vi "VISA MEMACC Write U8 vs U64.vi"() -> ()   [LabVIEW 2016]
uses:
  <vilib>/Platform/TimedLoop/XDataNode/timing_clust.ctl
  <vilib>/Platform/TimedLoop/XDataNode/nitl_modes.ctl
  <vilib>/Platform/TimedLoop/XDataNode/wakeup.ctl
  Source/GE 5565PIORC/GE 5565PIORC.lvclass/GE 5565PIORC.ctl
  Source/GE 5565PIORC/VIs/Block Operations/Allocate Single Block.vi
  Source/GE 5565PIORC/VIs/Registers/Local Configuration.LAS1RR.Address Range.Get.vi
  Source/GE 5565PIORC/VIs/Binary Operations/Align to 8-byte Boundary.vi
  Source/GE 5565PIORC/VIs/Binary Operations/Align to 16-byte Boundary.vi
  Source/GE 5565PIORC/VIs/Registers/Local Configuration.Get Register Offset.vi
  Source/GE 5565PIORC/GE 5565PIORC.lvclass
  <vilib>/platform/TimedLoop/XDataNode/XDataNode.xnode
  <vilib>/Platform/TimedLoop/XDataNode/XDNodeRunTimeDep.lvlib
panel:
  out "U64 Duration":dbl
  in  "U64s":i32
  out "U8 Duration":dbl
  in  "VISA resource name":refnum<visa-resource-name>
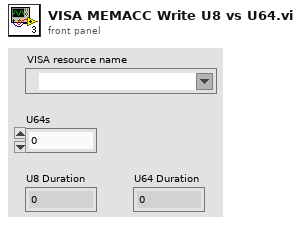
[diagram p1: front panel]
types:
  T1 = typedef "XDNodeRunTimeDep.lvlib/timing_clust.ctl" = cluster{"Expected End [f-1]":u64, "Actual End [f-1]":u64, "Finished Late? [f-1]":bool, "Expected End [i-1]":u64, "Actual End [i-1]":u64, "Finished Late? [i-1]":bool, "Expected Start [i]":u64, "Actual Start [i]":u64, "Expected Start [f]":u64, "Actual Start [f]":u64, "Source Name":string, "Structure Name":string, "Period":i64, "Deadline":i64, "Offset":i64, "Start":i64, "Priority":i32, "Timeout":i32, "Mode":T2, "Wakeup Reason":T3, "Error":errorcluster, "Source Type":string, "Secondary Source Type":string, "Global End Time":u64, "Global Start Time":u64, "Frame Duration":u64, "Iteration Duration":u64, "Assigned CPU":i32, "I/O Scan Engine Mode":u32}
  T2 = typedef "XDNodeRunTimeDep.lvlib/nitl_modes.ctl" = enum32{"No Change", "Process missed periods, maintain original phase", "Discard missed periods, maintain original phase", "Process missed periods, ignore original phase", "Discard missed periods, ignore original phase"}
  T3 = typedef "XDNodeRunTimeDep.lvlib/wakeup.ctl" = enum32{"Normal", "Aborted", "Asynchronous wakeup", "Timing source error", "Timed loop error", "Timeout"}
  T4 = typedef "GE 5565PIORC.lvclass/DMA Block Descriptor.ctl" = cluster{"descriptor ptr (VISA)":u32, "descriptor size":u32, "descriptor ptr (aligned)":u32, "data ptr (lower)":u32, "data ptr (upper)":u32, "data size":u32, "next descriptor ptr":u32}
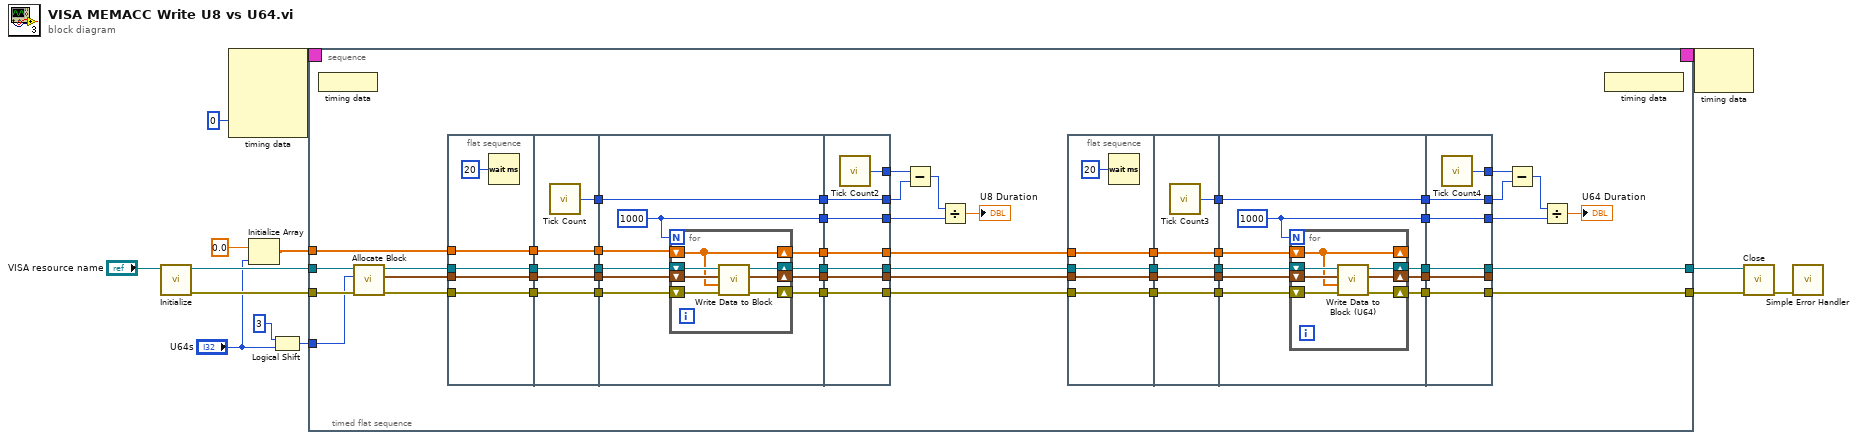
[diagram p0: block diagram]
diagram:
  n1 = call "Initialize.vi"("VISA resource name"="VISA resource name") -> ("error out"=w8:errorcluster, "GE 5565PIORC"=w9:refnum<class "GE 5565PIORC.lvclass">)  [unwired: 9 in]
  n2 = node-c288(0 ("Processor")) -> (w12:T1)  [unwired: 3 in]
  n3 = Initialize Array(0.0 ("element"), "U64s") -> (w1:dbl[])
  n4 = Logical Shift(y=i16 3, x="U64s") -> (x << y=w7:i32)
  n5 = timed-sequence {
    timing: w12 -> [_]
    timing-out: [_] -> w11
    tunnel: w9 -> [w17]
    tunnel: w8 -> [w20]
    tunnel: [w19] -> w4
    tunnel: w7 -> [w18]
    tunnel: [w16] -> w5
    tunnel: w1 -> [w15]
    n6 = timed-flat-sequence {
      tunnel: w20 -> [w45]
      tunnel: [w47] -> w19
      tunnel: w18 -> [w42]
      tunnel: w17 -> [w46]
      tunnel: [w28] -> w16
      tunnel: w15 -> [w27]
      n7 = node-c288() -> ()  [unwired: 1 in]
      n8 = call-poly "Allocate Block.vi"("error in (no error)"=w45, "size (bytes)"=w42, "GE 5565PIORC in"=w46) -> ("error out"=w43:errorcluster, "Block Descriptor"=w37:T4, "GE 5565PIORC out"=w44:refnum<class "GE 5565PIORC.lvclass">)  [unwired: 6 in]
      n9 = flat-sequence {
        tunnel: w44 -> [w108]
        tunnel: w43 -> [w107]
        tunnel: [w108] -> w67
        tunnel: [w107] -> w65
        tunnel: w37 -> [w106]
        tunnel: [w106] -> w36
        tunnel: w27 -> [w105]
        tunnel: [w105] -> w26
        tunnel: [w114] -> w72
        tunnel: [w113] -> w68
        tunnel: w67 -> [w113]
        tunnel: [w112] -> w66
        tunnel: w65 -> [w112]
        tunnel: w36 -> [w111]
        tunnel: [w111] -> w35
        tunnel: w26 -> [w110]
        tunnel: [w110] -> w25
        tunnel: w72 -> [w124]
        tunnel: [w124] -> w71
        tunnel: w68 -> [w121]
        tunnel: w66 -> [w120]
        tunnel: [w123] -> w64
        tunnel: [w122] -> w63
        tunnel: [w119] -> w41
        tunnel: w35 -> [w118]
        tunnel: [w117] -> w34
        tunnel: w25 -> [w116]
        tunnel: [w115] -> w24
        tunnel: [w138] -> w70
        tunnel: [w137] -> w69
        tunnel: w71 -> [w137]
        tunnel: w64 -> [w136]
        tunnel: [w136] -> w48
        tunnel: w63 -> [w135]
        tunnel: [w135] -> w61
        tunnel: w41 -> [w134]
        tunnel: [w134] -> w38
        tunnel: w34 -> [w133]
        tunnel: [w133] -> w33
        tunnel: w24 -> [w132]
        tunnel: [w132] -> w23
        frame #0 {
          n10 = Wait (ms)(milliseconds to wait=u32 20) -> ()  [unwired: 1 out]
        }
        frame #1 {
          n11 = call "Tick Count"() -> ("Tick Count(uSec)"=w114:u32)
        }
        frame #2 {
          w122 = 1000
          n12 = for {
            N: w122 -> [_]
            shift-right: [w130] -> w119
            shift-left: w121 -> [w131]
            shift-right: [w128] -> w123
            shift-left: w120 -> [w129]
            shift-right: [w127] -> w117
            shift-left: w118 -> [w126]
            shift-right: [w125] -> w115
            shift-left: w116 -> [w125]
            n13 = call "Write Data to Block.vi"("error in (no error)"=w129, "Data"=w125, "Block Descriptor"=w126, "GE 5565PIORC"=w131) -> ("error out"=w128:errorcluster, "Block Descriptor out"=w127:T4, "GE 5565PIORC out"=w130:refnum<class "GE 5565PIORC.lvclass">)  [unwired: 5 in]
          }
        }
        frame #3 {
          n14 = call "Tick Count2"() -> ("Tick Count(uSec)"=w138:u32)
        }
      }
      n15 = Subtract(x=w70, y=w69) -> (x-y=w62:u32)
      n16 = Divide(x=w62, y=w61) -> (x/y=→"U8 Duration":dbl)
      n17 = flat-sequence {
        tunnel: w48 -> [w76]
        tunnel: [w76] -> w59
        tunnel: [w75] -> w39
        tunnel: w38 -> [w75]
        tunnel: w33 -> [w74]
        tunnel: [w74] -> w32
        tunnel: w23 -> [w73]
        tunnel: [w73] -> w22
        tunnel: [w82] -> w58
        tunnel: [w81] -> w57
        tunnel: w59 -> [w81]
        tunnel: [w80] -> w40
        tunnel: w39 -> [w80]
        tunnel: w32 -> [w79]
        tunnel: [w79] -> w31
        tunnel: w22 -> [w78]
        tunnel: [w78] -> w21
        tunnel: w58 -> [w91]
        tunnel: [w91] -> w56
        tunnel: w57 -> [w86]
        tunnel: [w90] -> w55
        tunnel: [w89] -> w54
        tunnel: w40 -> [w88]
        tunnel: w31 -> [w87]
        tunnel: [w85] -> w30
        tunnel: [w84] -> w29
        tunnel: w21 -> [w83]
        tunnel: [w104] -> w53
        tunnel: [w103] -> w52
        tunnel: w56 -> [w103]
        tunnel: w55 -> [w102]
        tunnel: [w102] -> w47
        tunnel: w54 -> [w101]
        tunnel: [w101] -> w50
        tunnel: w30 -> [w99]
        tunnel: w29 -> [w100]
        tunnel: [w100] -> w28
        tunnel: [w99] -> _
        frame #0 {
          n18 = Wait (ms)(milliseconds to wait=u32 20) -> ()  [unwired: 1 out]
        }
        frame #1 {
          n19 = call "Tick Count3"() -> ("Tick Count(uSec)"=w82:u32)
        }
        frame #2 {
          w89 = 1000
          n20 = for {
            N: w89 -> [_]
            shift-right: [w97] -> w90
            shift-left: w86 -> [w98]
            shift-right: [w93] -> w84
            shift-left: w88 -> [w96]
            shift-right: [w94] -> w85
            shift-left: w87 -> [w95]
            shift-right: [w92] -> _
            shift-left: w83 -> [w92]
            n21 = call "Write Data to Block (U64).vi"("error in (no error)"=w98, "Data"=w92, "Block Descriptor"=w95, "GE 5565PIORC"=w96) -> ("error out"=w97:errorcluster, "Block Descriptor out"=w94:T4, "GE 5565PIORC out"=w93:refnum<class "GE 5565PIORC.lvclass">)  [unwired: 5 in]
          }
        }
        frame #3 {
          n22 = call "Tick Count4"() -> ("Tick Count(uSec)"=w104:u32)
        }
      }
      n23 = Subtract(x=w53, y=w52) -> (x-y=w51:u32)
      n24 = Divide(x=w51, y=w50) -> (x/y=→"U64 Duration":dbl)
      n25 = node-c288() -> ()  [unwired: 1 out]
    }
  }
  n26 = node-c288(w11) -> ()  [unwired: 1 out]
  n27 = call "Close.vi"("error in (no error)"=w4, "GE 5565PIORC in"=w5) -> ("error out"=w13:errorcluster)  [unwired: 8 in, 1 out]
  n28 = call <vilib>:"Simple Error Handler.vi"("error in (no error)"=w13) -> ()  [unwired: 4 in, 5 out]
